vi "FRCts20_Backend_Test_EventRoot_GET.vi"(8 "error in (no error)":errorcluster) -> (0 "error out":errorcluster, 1 "Time (ms)":u32, 2 "Status":string, 3 "Events":T1, 5 "Success":bool)   [LabVIEW 2013, in "FRCts20_Backend_TestCode.lvlib"]
uses:
  FRCts20_Backend_TestCode.lvlib
  FRCts20_Backend_API/FRCts20_Backend_API_EventRoot.ctl
  FRCts20_Backend_API/FRCts20_Backend_API_Command_EventRoot.ctl
  FRCts20_Backend_API/FRCts20_Backend_API_EventRoot.vi
  FRCts20_Backend_API/FRCts20_Backend_API.lvlib
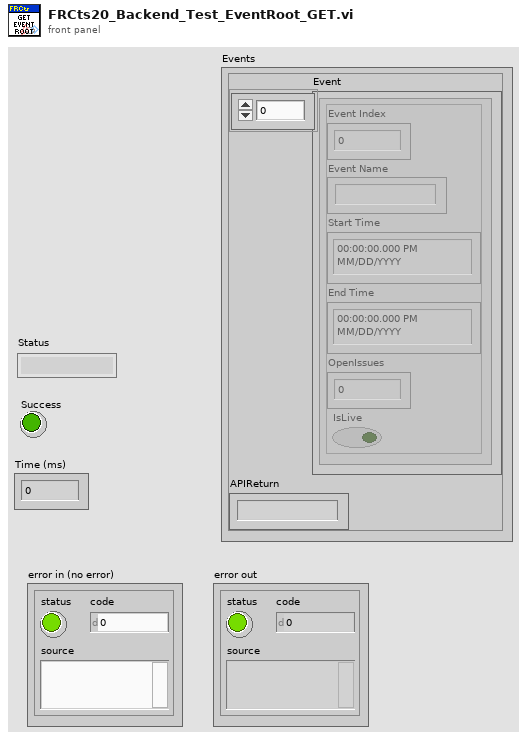
[diagram p1: front panel]
types:
  T1 = typedef "FRCts20_Backend_API.lvlib/FRCts20_Backend_API_EventRoot.ctl" = cluster{"Event":cluster{"Event Index":u32, "Event Name":string, "Start Time":timestamp, "End Time":timestamp, "OpenIssues":u8, "IsLive":bool}[], "APIReturn":string}
  T2 = typedef "FRCts20_Backend_API.lvlib/FRCts20_Backend_API_Command_EventRoot.ctl" = string
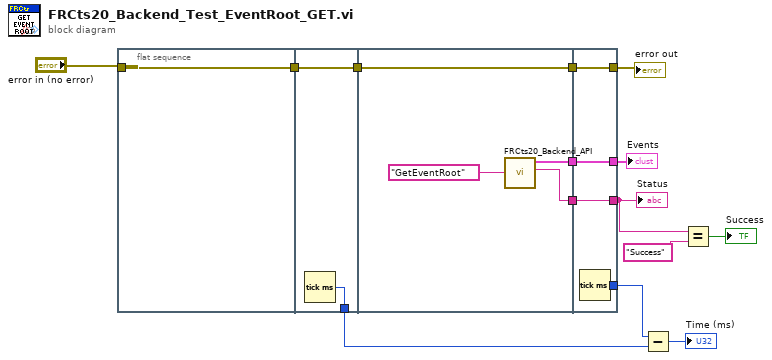
[diagram p0: block diagram]
diagram:
  n1 = flat-sequence {
    tunnel: "error in (no error)" -> [w15]
    tunnel: [w15] -> w14
    tunnel: [w17] -> w3
    tunnel: [w16] -> w13
    tunnel: w14 -> [w16]
    tunnel: [w21] -> w12
    tunnel: w13 -> [w21]
    tunnel: [w20] -> w11
    tunnel: [w19] -> w10
    tunnel: [w25] -> w4
    tunnel: [w24] -> w6
    tunnel: w12 -> [w24]
    tunnel: [w23] -> w1
    tunnel: w11 -> [w23]
    tunnel: [w22] -> w2
    tunnel: w10 -> [w22]
    frame #0 {
    }
    frame #1 {
      n2 = Tick Count (ms)() -> (millisecond timer value=w17:u32)
    }
    frame #2 {
      n3 = call-poly "FRCts20_Backend_API.vi"("Message"=T2 "GetEventRoot") -> ("Status"=w19:string, "EventRoot Out"=w20:T1)  [unwired: 8 in, 1 out]
    }
    frame #3 {
      n4 = Tick Count (ms)() -> (millisecond timer value=w25:u32)
    }
  }
  n5 = Subtract(x=w4, y=w3) -> (x-y=→"Time (ms)":u32)
  n6 = Equal?(x=w2, y="Success") -> (x = y?=→"Success":bool)
  "Status" <- w2
  "error out" <- w6
  "Events" <- w1
